vi "Actor Destroy Core.vi"(7 "Self Actor in":refnum<class "Self Actor.lvclass">, 11 "Destroying Self Actor State in":refnum<class "Destroying Self Actor State.lvclass">) -> (0 "error out":errorcluster)   [LabVIEW 2021, in "LVCAM.lvlib" / "Destroying Self Actor State.lvclass"]
uses:
  Destroying Self Actor State.lvclass
  Self Actor/Self Actor.lvclass
  Destroying Self Actor State.lvclass/Destroying Self Actor State.ctl
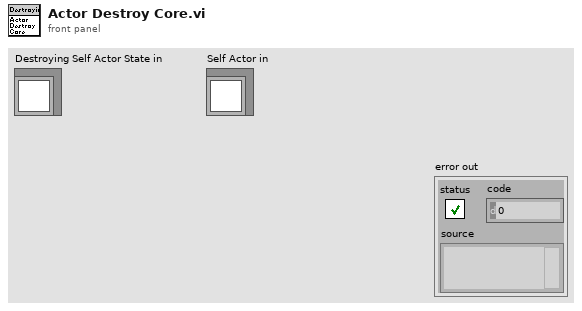
[diagram p1: front panel]
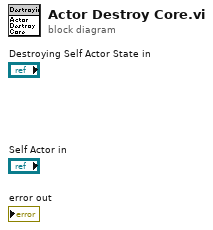
[diagram p0: block diagram]
diagram:
